vi "Read_binary_file.vi"(10 "Open path":path) -> (2 "message bitstream":i8[](array[numeric]))   [LabVIEW 2014]
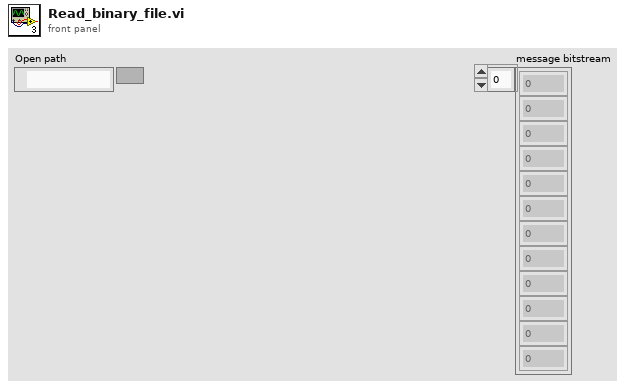
[diagram p1: front panel]
types:
  T1 = enum16{"big-endian, network order", "native, host order", "little-endian"}
  T2 = enum16{"open", "replace", "create", "open or create", "replace or create", "replace or create with confirmation"}
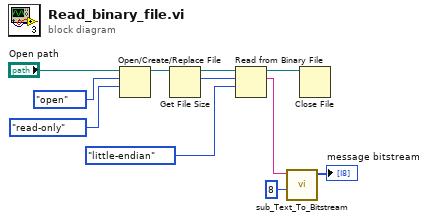
[diagram p0: block diagram]
diagram:
  n1 = Open/Create/Replace File(file path (use dialog)="Open path", operation (0:open)=T2."open", access (0:read/write)=enum16{"read/write", "read-only", "write-only"}."read-only") -> (refnum out=w9:refnum<file>)  [unwired: 3 in, 2 out]
  n2 = Get File Size(file=w9) -> (refnum out=w10:refnum<file>, size (in bytes)=w11:i64)  [unwired: 1 in, 1 out]
  n3 = Read from Binary File(9:T1."little-endian" ("byte order (0:big-endian, network order)"), 10:w11, 11:w10) -> (2:w3:string, 3:w5:refnum<file>)  [unwired: 3 in, 2 out]
  n4 = call "sub_Text_To_Bitstream.vi"("Packet\nMessage Length (bits)"=8 ("Packet\nMessage Length (bits)"), "text"=w3) -> ("message bitstream"=→"message bitstream":i8[])  [unwired: 7 in, 2 out]
  n5 = Close File(refnum=w5) -> ()  [unwired: 1 in, 2 out]
